vi "ke2002_conv_ABC_to_abd.vi"(0 "thermo":T1={"type"=enum."COMET Tx5xx (ethernet)", "comment"="", "tag"="", "refresh"=5.0, "IP"="", "port"=502, "VISA"="", "last readout"=timestamp(0 s since 1904-01-01), "TCP ref"=refnum, "VISA sess"="", "idn"="", "press"=0.0, "RH"=0.0, "temp"=0.0, "pres cor"=[], "RH cor"=[], "temp cor"=[], "try left"=0, "failed"=FALSE, "RTD set"=[], "RTD inv"=[], "range"=0.0, "net mode"=enum."MODBUS", "try fail"=enum."Stop trying - return NaN", "timeout [s]"=0.0, "max retries"=0, "sim t [deg]"=0.0} {"RTD inv" format="%.1f"; "RTD set" format="%.1f"; "temp cor" format="%.1f"; "RH cor" format="%.1f"; "pres cor" format="%.1f"; "refresh" min=0.1 max=1000.0 format="%.2f"}) -> (1 "R0":dbl, 2 "alpha":dbl, 3 "beta":dbl, 4 "delta":dbl)   [LabVIEW 2020]
uses:
  thermo.ctl
  thermo_types.ctl
  Thermometer Fail Action.ctl
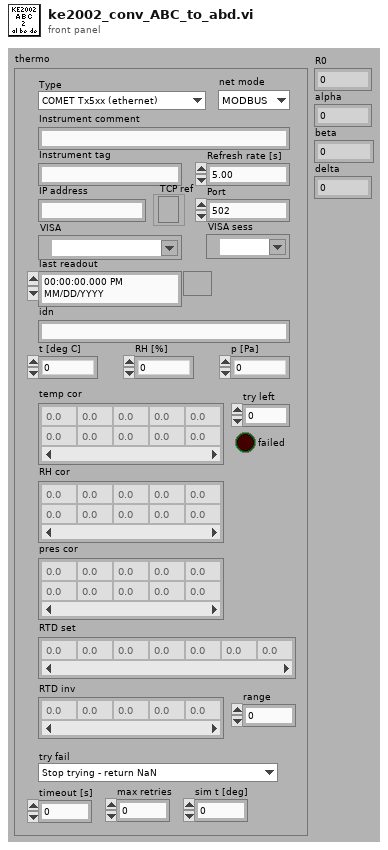
[diagram p1: front panel]
types:
  T1 = typedef "thermo.ctl" = cluster{"type":T2, "comment":string, "tag":string, "refresh":dbl, "IP":string, "port":u16, "VISA":refnum<visa-resource-name>, "last readout":timestamp, "TCP ref":refnum<k5>, "VISA sess":refnum<visa-resource-name>, "idn":string, "press":dbl, "RH":dbl, "temp":dbl, "pres cor":dbl[][], "RH cor":dbl[][], "temp cor":dbl[][], "try left":i32, "failed":bool, "RTD set":dbl[], "RTD inv":dbl[], "range":dbl, "net mode":enum16{"MODBUS", "HTTP"}, "try fail":T3, "timeout [s]":dbl, "max retries":i32, "sim t [deg]":dbl}
  T2 = typedef "thermo_types.ctl" = enum16{"Disabled", "Simulated", "COMET Tx5xx (ethernet)", "Keithley 2002 (GPIB) + RTD", "Agilent 344xx (GPIB) + RTD"}
  T3 = typedef "Thermometer Fail Action.ctl" = enum16{"Stop trying - keep last value", "Stop trying - return NaN", "Generate error - stop sweep"}
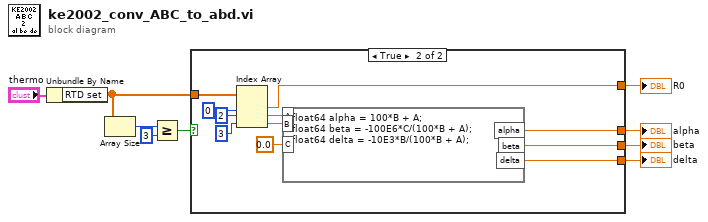
[diagram p0: block diagram]
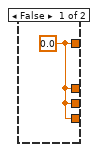
[diagram p2: hidden frame]
diagram:
  n1 = Unbundle By Name("thermo") -> ("RTD set"=w8:dbl[])
  n2 = Array Size(array=w8) -> (size(s)=w7:i32)
  n3 = Greater Or Equal?(x=w7, y=3) -> (x >= y?=w6:bool)
  n4 = case shown="True" w6 {
    tunnel: w8 -> [_ w21]
    tunnel: [w10 w14] -> w4
    tunnel: [w10 w13] -> w3
    tunnel: [w10 w12] -> w2
    tunnel: [w10 w11] -> w1
    frame False {
      w10 = 0.0 ("Numeric")
    }
    frame True {
      n5 = Index Array(array=w21, index #1=0 ("index"), index #2=2 ("index"), index #3=3 ("index")) -> (element #1=w14:dbl, element #2=w18:dbl, element #3=w17:dbl)
      n6 = formula code="float64 alpha = 100*B + A;\nfloat64 beta = -100E6*C/(100*B + A);\nfloat64 delta = -10E3*B/(100*B + A);"("A"=w18, "B"=w17, "C"=0.0 ("input variable")) -> ("alpha"=w13:dbl, "beta"=w12:dbl, "delta"=w11:dbl)
    }
  }
  "alpha" <- w3
  "beta" <- w2
  "delta" <- w1
  "R0" <- w4
